vi "UserInterfaceEventPattern 1.vi"() -> ()   [LabVIEW 2017]
doc: "Use this template to build a user interface event handler design pattern. Use this pattern for dialog boxes and other user interfaces. You also can create and execute user-defined events that the VI can handle the same way as user interface events."
uses:
  projects/lab/BOC/types/states_enum.ctl
  projects/lab/BOC/types/ui.ctl
  projects/lab/BOC/types/ui_buttons.ctl
panel:
  in  "Button 1":bool
  in  "stop":bool
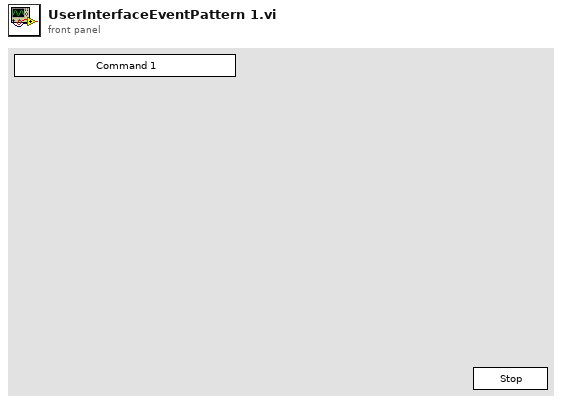
[diagram p1: front panel]
types:
  T1 = typedef "states_enum.ctl" = enum16{"init", "process", "exit"}
  T2 = typedef "ui.ctl" = cluster{"UI_buttons":T3, "Tab Control":refnum<vi>, "connect_button":refnum<vi>, "boc_type":enum16{"БОЦ-6", "БОЦ-12"}, "generator":refnum<visa-resource-name>, "voltmetr":refnum<visa-resource-name>}
  T3 = typedef "ui_buttons.ctl" = refnum<vi>[]
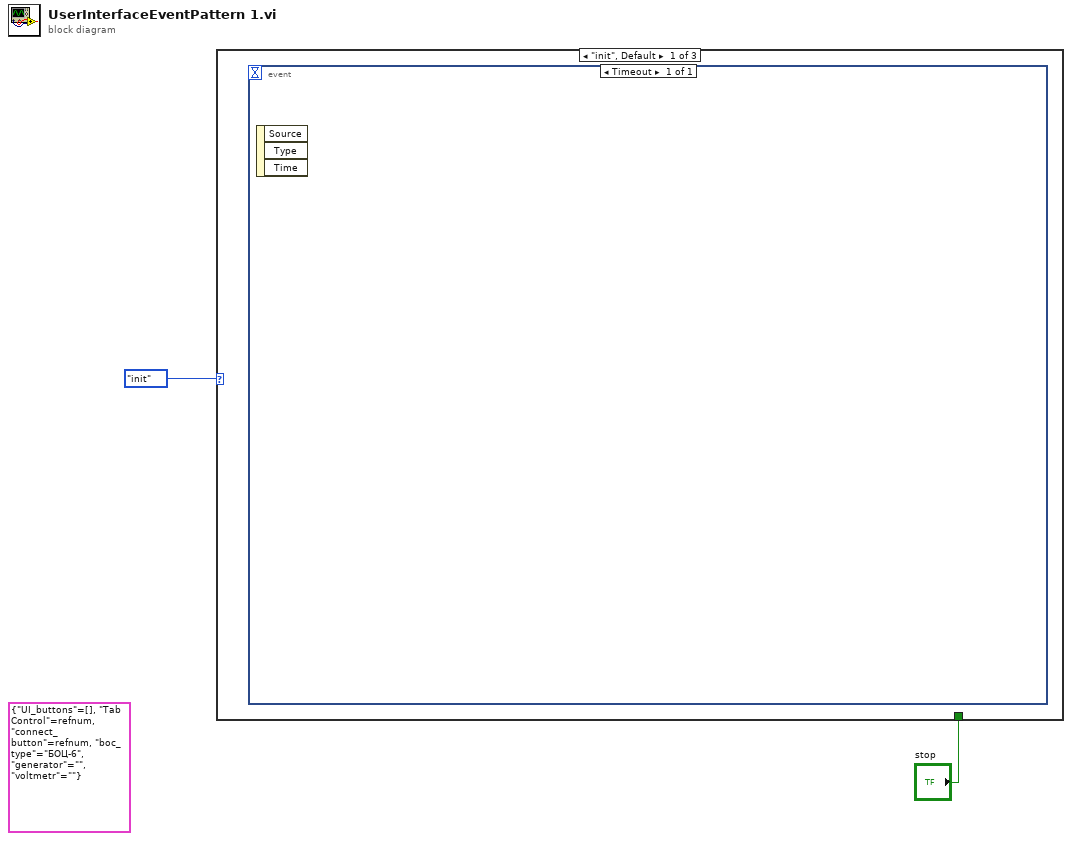
[diagram p0: block diagram]
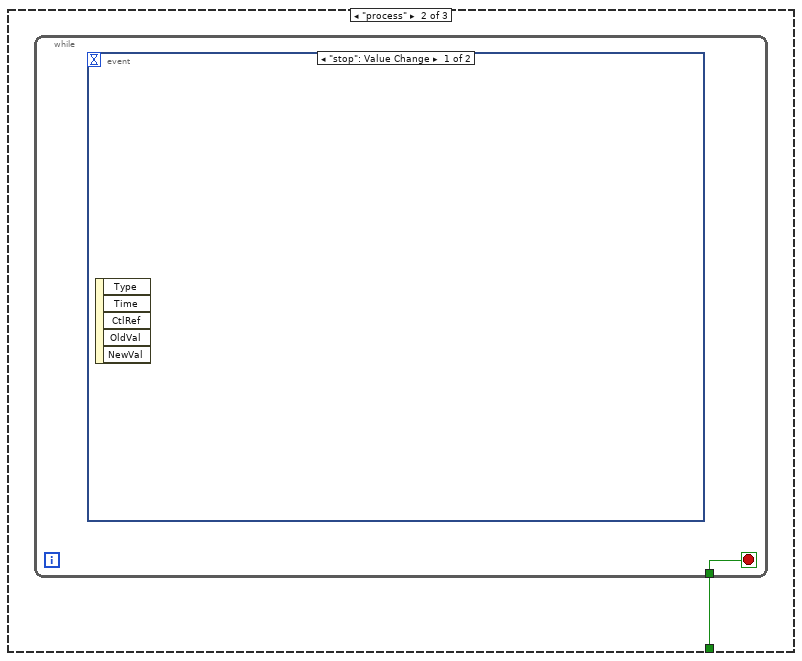
[diagram p2: hidden frame]
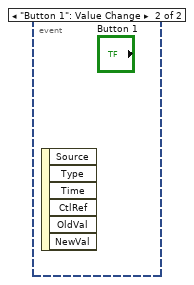
[diagram p3: hidden frame]
diagram:
  (unwired) T2 {"UI_buttons"=[], "Tab Control"=refnum, "connect_button"=refnum, "boc_type"=enum."БОЦ-6", "generator"="", "voltmetr"=""} ("UI")
  n1 = case shown="\"init\", Default" states_enum."init" ("Enum") {
    tunnel: "stop" -> [_ w3 _]
    frame "init", Default {
      n2 = event shown="[0] Timeout" {
        selector: _ -> [_]
        dyn-events: _ -> [_]
        timeout: _ -> [_]
        event Timeout {
          n3 = event-data() -> ()  [unwired: 1 in, 3 out]
        }
      }
    }
    frame "process" {
      n4 = while {
        tunnel: w3 -> [w4]
        stop <- w4 stop-if-true
        n5 = event shown="[0] \"stop\": Value Change" {
          selector: _ -> [_ _]
          dyn-events: _ -> [_ _]
          timeout: _ -> [_ _]
          event "stop": Value Change {
            n6 = event-data() -> ()  [unwired: 1 in, 5 out]
          }
          event "Button 1": Value Change {
            n7 = event-data() -> ()  [unwired: 1 in, 6 out]
          }
        }
      }
    }
    frame "exit" {
    }
  }
